vi "LeddarOpen.vi"(9 "Connection Mode":enum32{"INIT_FILE", "INIT_LIVE"}(radio), 11 "File path, USB name":string) -> (0 "Connection Mode Out":enum32{"INIT_FILE", "INIT_LIVE"}(radio), 1 "Success":bool, 2 "Event Callback":refnum<k27>, 3 "DeviceControl":refnum<k24>(container))   [LabVIEW 2012]
uses:
  C:/Program Files/LeddarTech/xtec/LeddarNET2.dll
panel:
  in  "DeviceControl":refnum<k24>(container)
  # "Example USB Address\nAC12345"
  # "Example File Path\nD:\\DEVICE-2013-06-19-14-07-16-824.ltl"
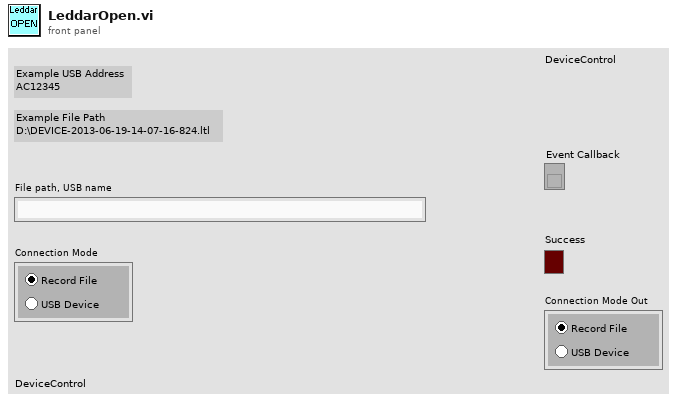
[diagram p1: front panel]
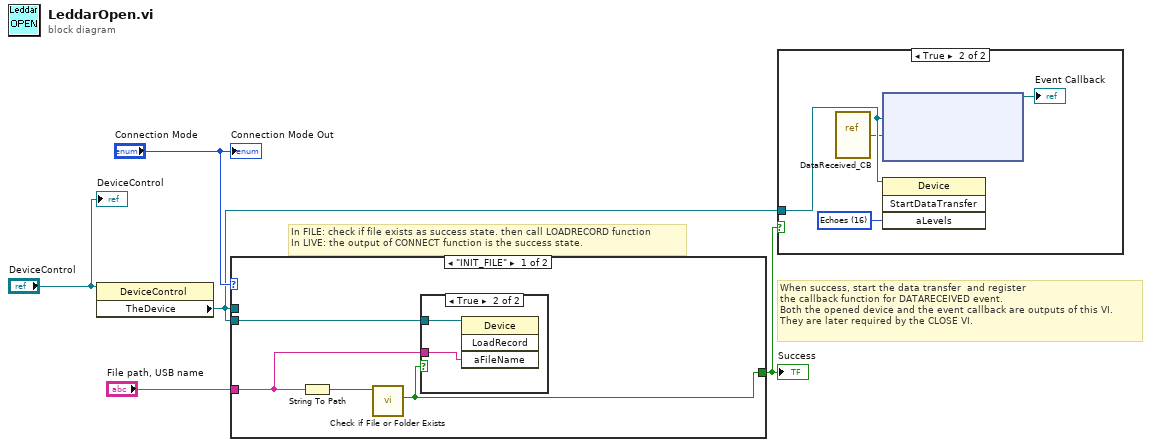
[diagram p0: block diagram]
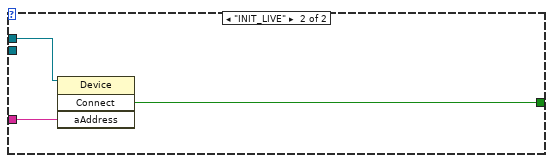
[diagram p4: hidden frame]
diagram:
  # "When success, start the data transfer  and register\nthe callback function for DATARECEIVED event.\nBoth the opened device and the event callback are outputs of this VI.\nThey are later required by the CLOSE VI."
  # "In FILE: check if file exists as success state. then call LOADRECORD function\nIn LIVE: the output of CONNECT function is the success state."
  n1 = property class="DeviceControl"(reference="DeviceControl") -> ("TheDevice"=w1:refnum<k24>)  [unwired: 1 in, 2 out]
  n2 = case shown="\"INIT_FILE\"" "Connection Mode" {
    tunnel: "File path, USB name" -> [w7 w14]
    tunnel: [w8 w13] -> w2
    tunnel: w1 -> [_ w12]
    tunnel: w1 -> [w9 _]
    frame "INIT_FILE" {
      n3 = String To Path(string=w7) -> (path=w6:path)
      n4 = call <vilib>:"Check if File or Folder Exists.vi"("path"=w6) -> ("file or folder exists?"=w8:bool)  [unwired: 8 in, 2 out]
      n5 = case shown="True" w8 {
        tunnel: w7 -> [_ w11]
        tunnel: w9 -> [_ w10]
        frame False {
        }
        frame True {
          n6 = invoke class="Device" method="LoadRecord"(reference=w10, "aFileName"=w11) -> ()  [unwired: 2 in, 4 out]
        }
      }
    }
    frame "INIT_LIVE" {
      n7 = invoke class="Device" method="Connect"(reference=w12, "aAddress"=w14) -> ("Connect"=w13:bool)  [unwired: 2 in, 3 out]
    }
  }
  "Success" <- w2
  n8 = case shown="True" w2 {
    tunnel: w1 -> [_ w16]
    frame False {
    }
    frame True {
      w17 = 16 items=["None"=0, "State"=2, "Echoes"=16] ("aLevels")
      n9 = vi-ref "DataReceived_CB.vi"() -> (w15:refnum<vi>)
      n10 = node(w16, w15) -> (→"Event Callback":refnum<k27>)  [unwired: 3 in, 1 out]
      n11 = invoke class="Device" method="StartDataTransfer"(reference=w16, "aLevels"=w17) -> ()  [unwired: 2 in, 4 out]
    }
  }
  "DeviceControl" <- "DeviceControl"
  "Connection Mode Out" <- "Connection Mode"
